vi "ProdaNG.Example.GetTestSteps3.vi"() -> ()   [LabVIEW 2015]
uses:
  Controls/ProdaNG.Process.ctl
  Controls/ProdaNG.ProcessStep.ctl
  Controls/ProdaNG.TestStep.ctl
panel:
  out "Process Steps":cluster{"ProcessStep":T1, "TestSteps":T2[]}[](array[cluster])
  out "Process":T3
  out "error out":errorcluster {"code" format="%.2f"}
  in  "Connection string":string="lcptb/lcptb@WCQPRO"
  in  "System":string="lin"
  in  "Wabco Number":string="0000001230"
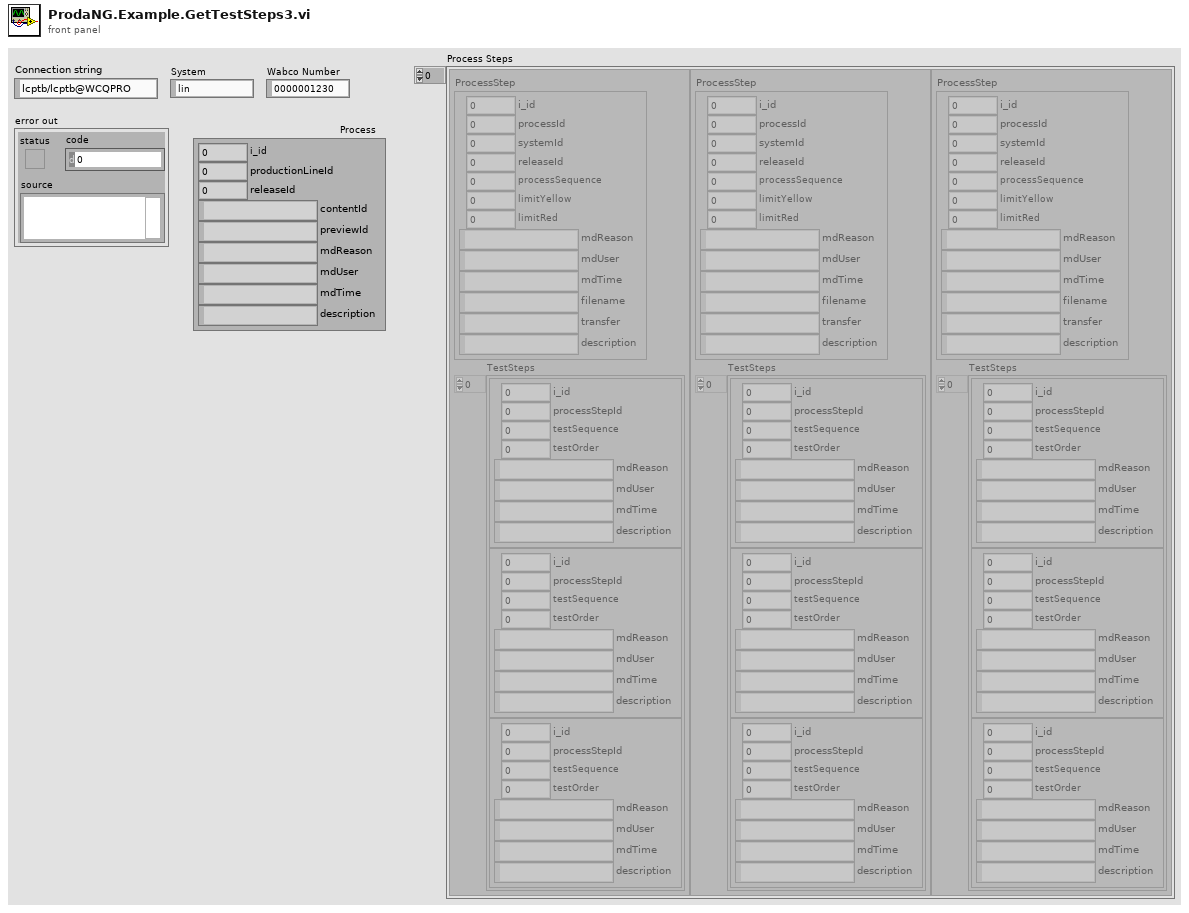
[diagram p1: front panel]
types:
  T1 = typedef "ProdaNG.ProcessStep.ctl" = cluster{"i_id":i32, "processId":i32, "systemId":i32, "releaseId":i32, "processSequence":i32, "limitYellow":dbl, "limitRed":dbl, "mdReason":string, "mdUser":string, "mdTime":string, "filename":string, "transfer":string, "description":string}
  T2 = typedef "ProdaNG.TestStep.ctl" = cluster{"i_id":i32, "processStepId":i32, "testSequence":i32, "testOrder":i32, "mdReason":string, "mdUser":string, "mdTime":string, "description":string}
  T3 = typedef "ProdaNG.Process.ctl" = cluster{"i_id":i32, "productionLineId":i32, "releaseId":i32, "contentId":string, "previewId":string, "mdReason":string, "mdUser":string, "mdTime":string, "description":string}
  T4 = typedef "ProdaNG.Identification.ctl" = cluster{"processId":i32, "systemId":i32, "processStepId":i32, "wabcoPartId":i32}
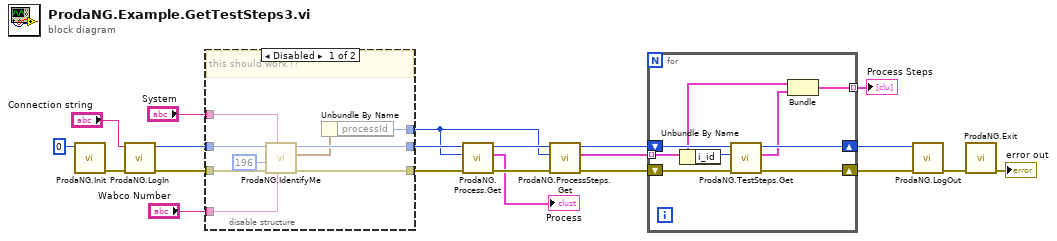
[diagram p0: block diagram]
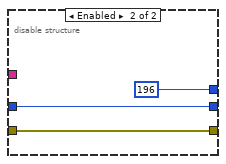
[diagram p2: hidden frame]
diagram:
  n1 = call "ProdaNG.Init.vi"("numContexts (0: unlimited)"=0 ("numContexts")) -> ("error out"=w21:errorcluster)  [unwired: 10 in]
  n2 = call "ProdaNG.LogIn.vi"("error in"=w21, "ConnectionString"="Connection string") -> ("error out"=w13:errorcluster, "dbHandle"=w14:i32)  [unwired: 7 in, 1 out]
  n3 = disable-structure shown="Disabled" {
    disable-tunnel: "System" -> [w30 _]
    disable-tunnel: "Wabco Number" -> [w29 _]
    disable-tunnel: w14 -> [w28 w33]
    disable-tunnel: w13 -> [w27 w32]
    disable-tunnel: [w25 w33] -> w12
    disable-tunnel: [w24 w32] -> w8
    disable-tunnel: [w22 196 ("processId")] -> w1
    frame Disabled {
      # "this should work !?"
      n4 = call "ProdaNG.IdentifyMe.vi"("wabcoNumber"=w29, "systemName"=w30, "error in"=w27, "processSequence"=196, "dbHandleIn"=w28) -> ("error out"=w24:errorcluster, "Identification"=w23:T4, "dbHandle"=w25:i32)  [unwired: 4 in]
      n5 = Unbundle By Name(w23) -> ("processId"=w22:i32)
    }
    frame Enabled {
    }
  }
  n6 = call "ProdaNG.Process.Get.vi"("error in (no error)"=w8, "processId"=w1, "dbHandleIn"=w12) -> ("error out"=w7:errorcluster, "Process"=→"Process":T3, "dbHandle"=w11:i32)  [unwired: 5 in, 1 out]
  n7 = call "ProdaNG.ProcessSteps.Get.vi"("error in (no error)"=w7, "processId"=w1, "dbHandleIn"=w11) -> ("error out"=w6:errorcluster, "ProcSteps"=w3:T1[], "dbHandle"=w10:i32)  [unwired: 6 in]
  n8 = for {
    shift-right: [w40] -> w9
    shift-left: w10 -> [w41]
    shift-right: [w38] -> w5
    shift-left: w6 -> [w39]
    tunnel: w3 -> [w35] mode=indexing
    tunnel: [w34] -> w2 mode=indexing
    n9 = Unbundle By Name(w35) -> ("i_id"=w37:i32)
    n10 = call "ProdaNG.TestSteps.Get.vi"("error in (no error)"=w39, "processStepId"=w37, "dbHandleIn"=w41) -> ("error out"=w38:errorcluster, "TestSteps"=w36:T2[], "dbHandle"=w40:i32)  [unwired: 6 in]
    n11 = Bundle("ProcessStep"=w35, "TestSteps"=w36) -> (w34:cluster{"ProcessStep":T1, "TestSteps":T2[]})  [unwired: 1 in]
  }
  "Process Steps" <- w2
  n12 = call "ProdaNG.LogOut.vi"("error in"=w5, "dbHandleIn"=w9) -> ("error out"=w16:errorcluster)  [unwired: 9 in]
  n13 = call "ProdaNG.Exit.vi"("error in (no error)"=w16) -> ("error out"=→"error out":errorcluster)  [unwired: 10 in]
